vi "Basic Write and Read Example.vi"() -> ()   [LabVIEW 2018]
uses:
  <vilib>/NI Veristand/Execution/Workspace/NI_VS Workspace ExecutionAPI.lvlib
panel:
  out "Valid Measurements?":bool
  out "error out":errorcluster
  in  "error in (no error)":errorcluster
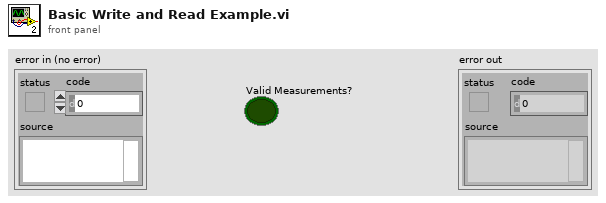
[diagram p1: front panel]
types:
  T1 = typedef "NI_VS Workspace ExecutionAPI.lvlib/WorkspaceAPI.ctl" = refnum<k24>
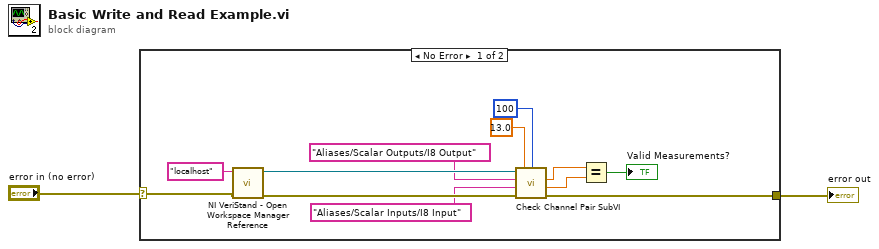
[diagram p0: block diagram]
diagram:
  n1 = case shown="No Error" "error in (no error)" {
    selector: "error in (no error)" -> [w14 w15]
    tunnel: [w10 w15] -> w1
    frame No Error {
      n2 = call <vilib>:"NI VeriStand - Open Workspace Manager Reference.vi"("error in (no error)"=w14, "Gateway IP Address (\"\": localhost)"="localhost" ("Gateway IP Address (\"\": localhost)")) -> ("error out"=w11:errorcluster, "WorkspaceManager"=w9:T1)  [unwired: 8 in]
      n3 = call "Check Channel Pair SubVI.vi"("milliseconds to wait"=u32 100, "Test Value"=13.0 ("Value"), "error in (no error)"=w11, "Input Channel"="Aliases/Scalar Inputs/I8 Input" ("Channel"), "Output Channel"="Aliases/Scalar Outputs/I8 Output" ("Channel"), "WorkspaceManager in"=w9) -> ("error out"=w10:errorcluster, "InputChannel Value"=w5:dbl, "OutputChannel Value"=w6:dbl)  [unwired: 2 in, 1 out]
      n4 = Equal?(x=w6, y=w5) -> (x = y?=→"Valid Measurements?":bool)
    }
    frame Error {
    }
  }
  "error out" <- w1
